vi "Set Current.vi"(8 "error in (no error)":errorcluster, 10 "Current [mA]":dbl, 11 "Simple Device in":refnum<class "Simple Device.lvclass">) -> (0 "error out":errorcluster, 3 "Simple Device out":refnum<class "Simple Device.lvclass">)   [LabVIEW 2021, in "Simple Device.lvclass"]
uses:
  Simple Device.lvclass
  Simple Device.lvclass/Simple Device.ctl
  TALOS/TALOS_PPL.lvlibp
  Libraries/Virtual Device Simulator/DeviceSim.lvlibp/DeviceReference/Simple  Virtual Device.lvclass
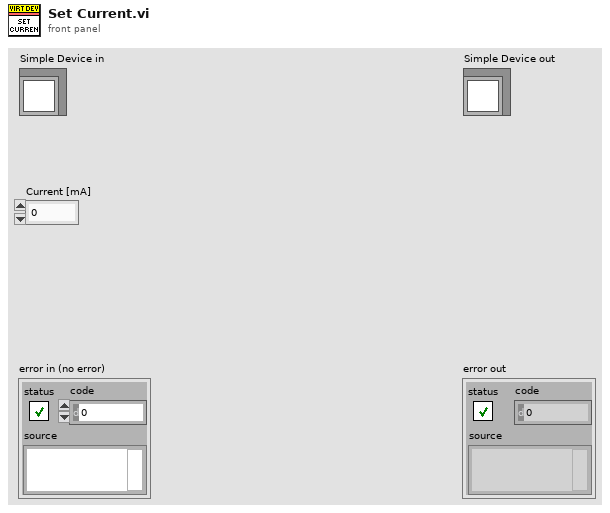
[diagram p1: front panel]
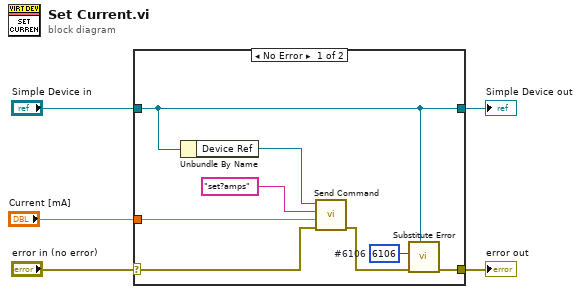
[diagram p0: block diagram]
diagram:
  n1 = case shown="No Error" "error in (no error)" {
    selector: "error in (no error)" -> [w9 w15]
    tunnel: [w13 w15] -> w4
    tunnel: [w12 w14] -> w2
    tunnel: "Simple Device in" -> [w12 w14]
    tunnel: "Current [mA]" -> [w8 _]
    frame No Error {
      w11 = 6106  # #6106
      n2 = Unbundle By Name(w12) -> ("Device Ref"=w6:refnum<data-value>)
      n3 = call "Send Command.vi"("error in (no error)"=w9, "Data"=w8, "Command"="set?amps", "Device Ref in"=w6) -> ("error out"=w10:errorcluster)  [unwired: 5 in, 2 out]
      n4 = call "Substitute Error.vi"("LabVIEW Object"=w12, "error in (no error)"=w10, "Error Code"=w11) -> ("error out"=w13:errorcluster)  [unwired: 8 in]
    }
    frame Error {
    }
  }
  "error out" <- w4
  "Simple Device out" <- w2
